vi "Variable globale.vi"() -> ()   [LabVIEW 2020]
uses:
  File et notificateur/File et notification.ctl
  TypeDef/Data Event Sequenceur.ctl
  TypeDef/Liste Event Sequenceur.ctl
  TypeDef/Liste Fonction appelante.ctl
  Tache Generation Historique/Type DEF/Data Event Historique.ctl
  Tache Generation Historique/Type DEF/Liste Event Historique.ctl
  Type DEF/Commande Selection produit en cours.ctl
  TypeDef/Commande Variable Global.ctl
  Type DEF/Commande Variables Programme.ctl
  Type DEF/Commande tableau Resultat.ctl
  Instrument/BLE/Comande Variable Globale BLE.ctl
  Drivers/BLE/type_def/connection_status_bundle.ctl
  Drivers/BLE/type_def/address_type.ctl
  Type DEF/Commande Event Demande Op.ctl
  Type DEF/Commande Event Demande Autotest.ctl
  Type DEF/Commande Action Lecture RS Bridge.ctl
  Type DEF/Commande Event Saisie Op.ctl
  TypeDef/Liste fonction Saisie Operateur.ctl
  Type DEF/Commande Event Affiche Result.ctl
  Fonction/Shielding Box/Action.ctl
  TypeDef/Adresse IHM.ctl
panel:
  out "First Test":bool
  out "File et Queue":T1
  out "liste trouvée":string[](array[string])
  # "Application"
  # "Sequenceur"
  # "Data"
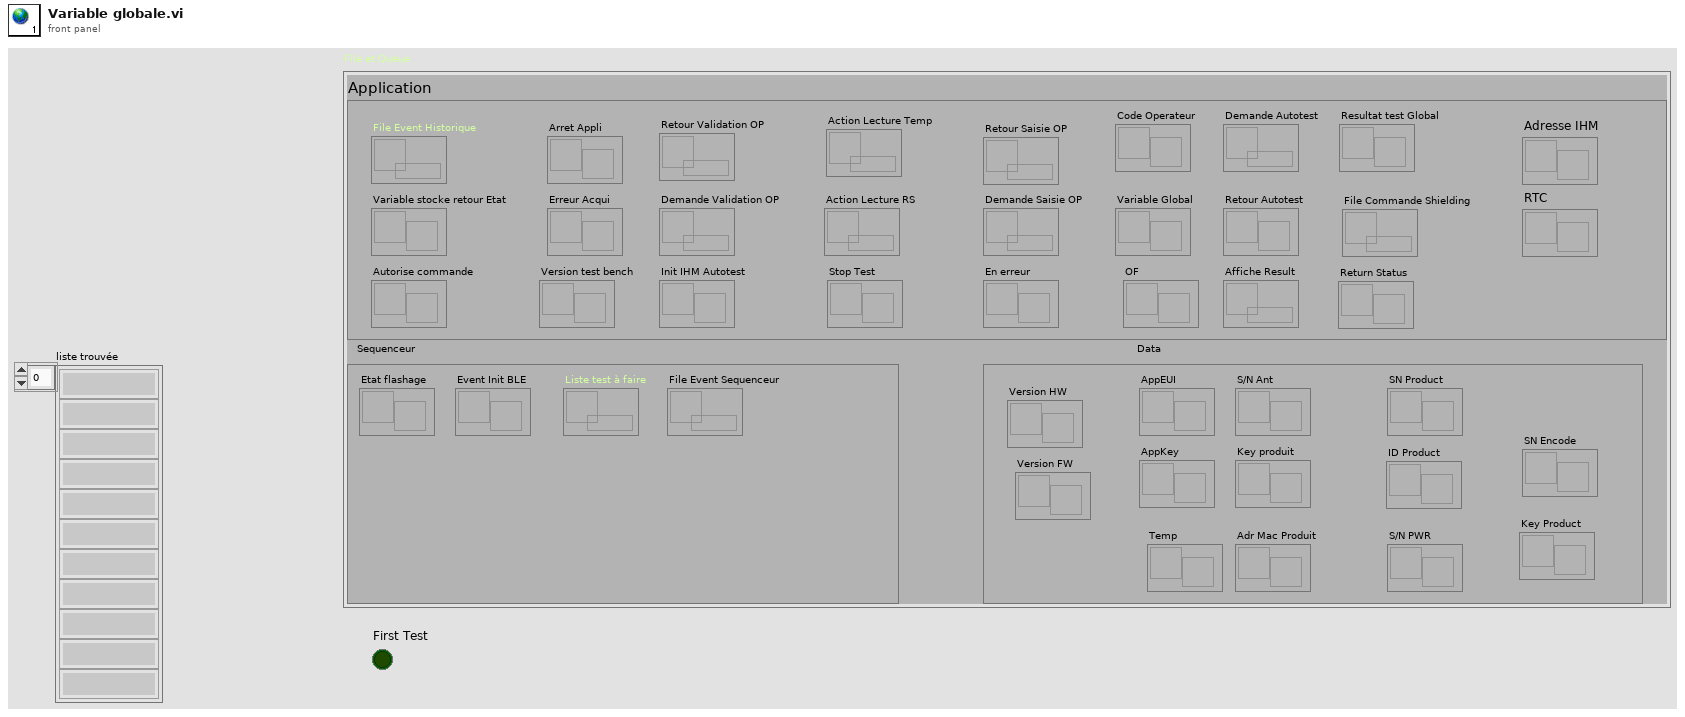
[diagram p1: front panel]
types:
  T1 = typedef "File et notification.ctl" = cluster{"Arret Appli":refnum<notifier>, "Erreur Acqui":refnum<notifier>, "File Event Sequenceur":refnum<queue>, "Liste test à faire":refnum<queue>, "File Event Historique":refnum<queue>, "Variable Global":refnum<notifier>, "Variable stocke retour Etat":refnum<notifier>, "Retour Validation OP":refnum<queue>, "Demande Validation OP":refnum<queue>, "Retour Autotest":refnum<notifier>, "Demande Autotest":refnum<queue>, "Adr Mac Produit":refnum<notifier>, "Autorise commande":refnum<notifier>, "Event Init BLE":refnum<notifier>, "Action Lecture RS":refnum<queue>, "Key produit":refnum<notifier>, "Retour Saisie OP":refnum<queue>, "Demande Saisie OP":refnum<queue>, "Etat flashage":refnum<notifier>, "Code Operateur":refnum<notifier>, "Resultat test Global":refnum<notifier>, "Stop Test":refnum<notifier>, "Init IHM Autotest":refnum<notifier>, "Version test bench":refnum<notifier>, "SN Product":refnum<notifier>, "En erreur":refnum<notifier>, "Affiche Result":refnum<queue>, "S/N PWR":refnum<notifier>, "AppEUI":refnum<notifier>, "Action Lecture Temp":refnum<queue>, "Temp":refnum<notifier>, "AppKey":refnum<notifier>, "OF":refnum<notifier>, "File Commande Shielding":refnum<queue>, "Return Status":refnum<notifier>, "ID Product":refnum<notifier>, "Version FW":refnum<notifier>, "Version HW":refnum<notifier>, "Adresse IHM":refnum<notifier>, "RTC":refnum<notifier>, "S/N Ant":refnum<notifier>, "SN Encode":refnum<notifier>, "Key Product":refnum<notifier>}
diagram:
